vi "ExSubInitOnlineGlobals.vi"   [LabVIEW 2010]
uses:
  GlobalFlipFlag.vi
  GlobalReverseFlag.vi
  GlobalIBackImgHndl.vi
  GlobalIFlatImgHndl.vi
  GlobalInitializeFlag.vi
  GlobalExposure.vi
  GlobalTimingMode.vi
  GlobalFramesToStr.vi
  GlobalAcquireFocusFlag.vi
  GlobalFullBin.vi
  GlobalBin2x.vi
  GlobalUserBin.vi
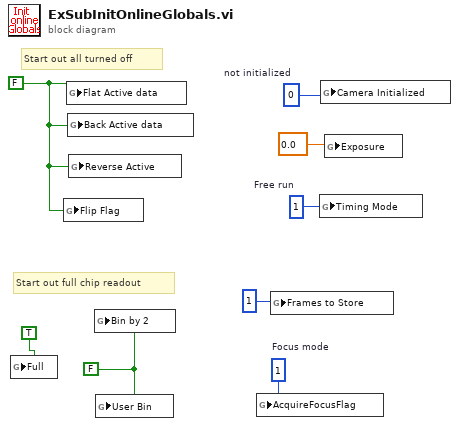
[diagram p0: block diagram]
diagram:
  w2 = FALSE
  w3 = 1  # Focus mode
  w5 = 1  # Free run
  w7 = 0  # not initialized
  w8 = FALSE
  # "Start out full chip readout"
  # "Start out all turned off"
  n1 = global write "GlobalFullBin.vi" "Full"(TRUE) -> ()
  n2 = global write "GlobalFlipFlag.vi" "Flip Flag"(w8) -> ()
  n3 = global write "GlobalIFlatImgHndl.vi" "Flat Active data"(w8) -> ()
  n4 = global write "GlobalIBackImgHndl.vi" "Back Active data"(w8) -> ()
  n5 = global write "GlobalReverseFlag.vi" "Reverse Active"(w8) -> ()
  n6 = global write "GlobalBin2x.vi" "Bin by 2"(w2) -> ()
  n7 = global write "GlobalUserBin.vi" "User Bin"(w2) -> ()
  n8 = global write "GlobalAcquireFocusFlag.vi" "AcquireFocusFlag"(w3) -> ()
  n9 = global write "GlobalFramesToStr.vi" "Frames to Store"(1) -> ()
  n10 = global write "GlobalTimingMode.vi" "Timing Mode"(w5) -> ()
  n11 = global write "GlobalInitializeFlag.vi" "Camera Initialized"(w7) -> ()
  n12 = global write "GlobalExposure.vi" "Exposure"(0.0) -> ()
